vi "Get Descriptor.vi"(0 "VISA resource name":refnum<visa-resource-name>, 5 "Source (0: Channel 1)":u16(ring) items=["Channel 1", "Channel 2", "Channel 3", "Channel 4", "Memory 1", "Memory 2", "Memory 3", "Memory 4", "Function 1", "Function 2", "Function 3", "Function 4", "Function 5", "Function 6", "Function 7", "Function 8", "Other"], 7 "Custom Source ID":string, 11 "error in (no error)":errorcluster) -> (1 "First Valid Point":i32, 2 "Last Valid Point":i32, 3 "Horizontal interval":sgl, 4 "VISA resource name out":refnum<visa-resource-name>, 6 "Vertical gain":sgl, 8 "Horizontal Offset":dbl, 10 "Vertical offset":sgl, 12 "Number Of Data Points":i32, 13 "Trigger Time":T1, 14 "Command type":i16, 15 "error out":errorcluster)   [LabVIEW 2013, in "LeCroy Wave Series.lvlib"]
doc: "Get basic information about acquisition waveform from specified channel."
uses:
  <instrlib>/LeCroy Wave Series/LeCroy Wave Series.lvlib
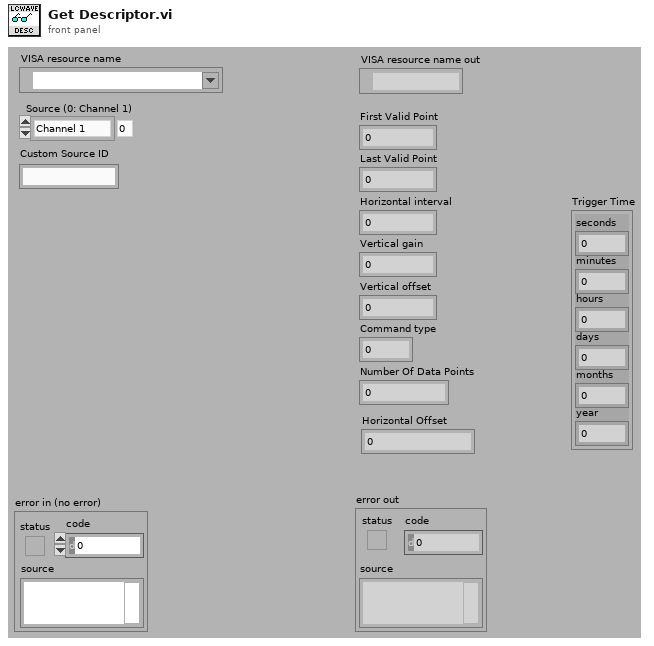
[diagram p1: front panel]
types:
  T1 = cluster{"seconds":dbl, "minutes":u8, "hours":u8, "days":u8, "months":u8, "year":u16}
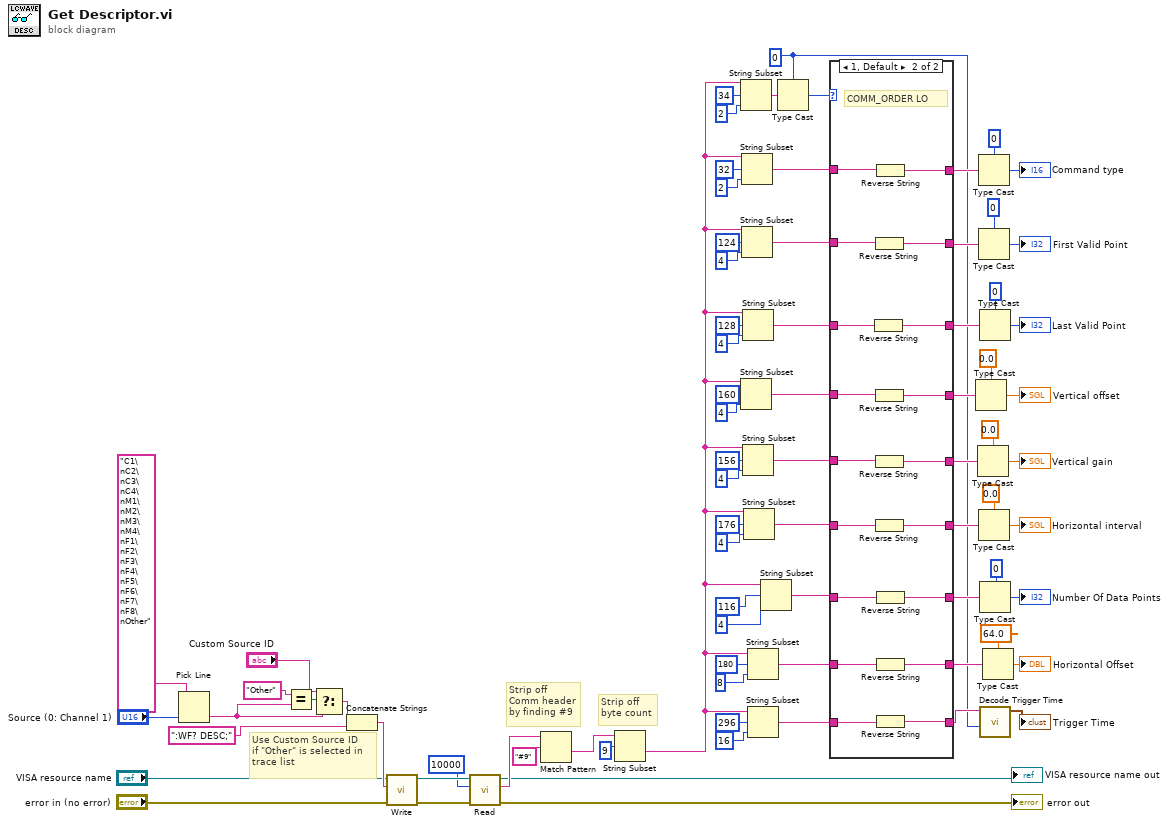
[diagram p0: block diagram]
diagram:
  w1 = i16 0
  # "Use Custom Source ID\nif \"Other\" is selected in \ntrace list"
  # "Strip off byte count"
  # "Strip off\nComm header\nby finding #9"
  n1 = Pick Line(multi-line string="C1\nC2\nC3\nC4\nM1\nM2\nM3\nM4\nF1\nF2\nF3\nF4\nF5\nF6\nF7\nF8\nOther", line index="Source (0: Channel 1)") -> (output string=w15:string)  [unwired: 1 in]
  n2 = Equal?(x="Other", y=w15) -> (x = y?=w17:bool)
  n3 = Select(t="Custom Source ID", s=w17, f=w15) -> (s? t:f=w14:string)
  n4 = Concatenate Strings(w14, ":WF? DESC;" ("write buffer")) -> (w24:string)
  n5 = call <instrlib>:"Write.vi"("error in (no error)"="error in (no error)", "Write Buffer"=w24, "VISA resource name"="VISA resource name") -> ("error out"=w30:errorcluster, "VISA resource name out"=w22:refnum<visa-resource-name>)  [unwired: 6 in, 1 out]
  n6 = call <instrlib>:"Read.vi"("error in (no error)"=w30, "Byte Count"=u32 10000, "VISA resource name"=w22) -> ("error out"=→"error out":errorcluster, "Read Buffer"=w20:string, "VISA resource name out"=→"VISA resource name out":refnum<visa-resource-name>)  [unwired: 5 in, 1 out]
  n7 = Match Pattern(string=w20, regular expression="#9") -> (after substring=w31:string)  [unwired: 1 in, 3 out]
  n8 = String Subset(string=w31, offset (0)=9 ("length (rest)")) -> (substring=w5:string)  [unwired: 1 in]
  n9 = String Subset(string=w5, offset (0)=34, length (rest)=2 ("length (rest)")) -> (substring=w59:string)
  n10 = String Subset(string=w5, offset (0)=160, length (rest)=4 ("length (rest)")) -> (substring=w74:string)
  n11 = String Subset(string=w5, offset (0)=32, length (rest)=2 ("length (rest)")) -> (substring=w49:string)
  n12 = String Subset(string=w5, offset (0)=124, length (rest)=4 ("length (rest)")) -> (substring=w55:string)
  n13 = String Subset(string=w5, offset (0)=128, length (rest)=4 ("length (rest)")) -> (substring=w37:string)
  n14 = String Subset(string=w5, offset (0)=156, length (rest)=4 ("length (rest)")) -> (substring=w68:string)
  n15 = String Subset(string=w5, offset (0)=176, length (rest)=4 ("length (rest)")) -> (substring=w63:string)
  n16 = String Subset(string=w5, offset (0)=180, length (rest)=8 ("length")) -> (substring=w11:string)
  n17 = String Subset(string=w5, offset (0)=296, length (rest)=16 ("length (rest)")) -> (substring=w4:string)
  n18 = String Subset(string=w5, offset (0)=116, length (rest)=4 ("length (rest)")) -> (substring=w45:string)
  n19 = Type Cast(type=w1, x=w59) -> (*(type *) &x=w58:i16)
  n20 = case shown="1, Default" w58 {
    tunnel: [w88 w106] -> w75
    tunnel: w74 -> [w88 w105]
    tunnel: [w87 w104] -> w69
    tunnel: w68 -> [w87 w103]
    tunnel: [w86 w102] -> w64
    tunnel: w63 -> [w86 w101]
    tunnel: w55 -> [w85 w100]
    tunnel: [w85 w99] -> w52
    tunnel: w49 -> [w84 w94]
    tunnel: [w84 w93] -> w47
    tunnel: [w83 w97] -> w44
    tunnel: w45 -> [w83 w98]
    tunnel: w37 -> [w82 w96]
    tunnel: [w82 w95] -> w36
    tunnel: w11 -> [w81 w92]
    tunnel: [w81 w91] -> w10
    tunnel: w4 -> [w80 w90]
    tunnel: [w80 w89] -> w3
    frame 0 {
      # "COMM_ORDER HI"
    }
    frame 1, Default {
      # "COMM_ORDER LO"
      n21 = Reverse String(1:w96) -> (0:w95:string)
      n22 = Reverse String(1:w100) -> (0:w99:string)
      n23 = Reverse String(1:w105) -> (0:w106:string)
      n24 = Reverse String(1:w103) -> (0:w104:string)
      n25 = Reverse String(1:w101) -> (0:w102:string)
      n26 = Reverse String(1:w94) -> (0:w93:string)
      n27 = Reverse String(1:w98) -> (0:w97:string)
      n28 = Reverse String(1:w92) -> (0:w91:string)
      n29 = Reverse String(1:w90) -> (0:w89:string)
    }
  }
  n30 = Type Cast(type=sgl 0.0, x=w75) -> (*(type *) &x=→"Vertical offset":sgl)
  n31 = Type Cast(type=sgl 0.0, x=w69) -> (*(type *) &x=→"Vertical gain":sgl)
  n32 = Type Cast(type=i16 0, x=w47) -> (*(type *) &x=→"Command type":i16)
  n33 = Type Cast(type=0, x=w52) -> (*(type *) &x=→"First Valid Point":i32)
  n34 = Type Cast(type=sgl 0.0, x=w64) -> (*(type *) &x=→"Horizontal interval":sgl)
  n35 = Type Cast(type=0, x=w36) -> (*(type *) &x=→"Last Valid Point":i32)
  n36 = Type Cast(type=0, x=w44) -> (*(type *) &x=→"Number Of Data Points":i32)
  n37 = call <instrlib>:"Decode Trigger Time.vi"("Comm_order"=w1, "Trigger_time string"=w3) -> ("Trigger Time"=→"Trigger Time":T1)  [unwired: 8 in]
  n38 = Type Cast(type=64.0, x=w10) -> (*(type *) &x=→"Horizontal Offset":dbl)
